vi "Convert Time to UTC String.vi"(11 "timestamp":timestamp) -> (3 "UTC string":string)   [LabVIEW 2019, in "CAN Stream Support Workspace Shared.lvlib"]
uses:
  CAN Stream Support Workspace Shared.lvlib
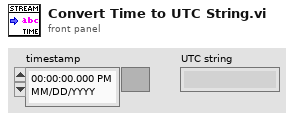
[diagram p1: front panel]
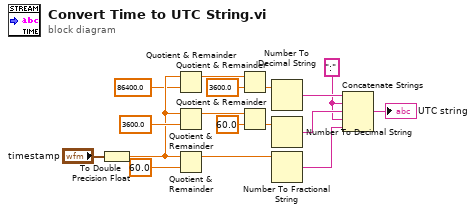
[diagram p0: block diagram]
diagram:
  w3 = ":" ("string")
  n1 = To Double Precision Float(number="timestamp") -> (double precision float=w14:dbl)
  n2 = Quotient & Remainder(x=w14, y=86400.0) -> (x-y*floor(x/y)=w10:dbl)  [unwired: 1 out]
  n3 = Quotient & Remainder(x=w14, y=3600.0) -> (x-y*floor(x/y)=w11:dbl)  [unwired: 1 out]
  n4 = Quotient & Remainder(x=w14, y=60.0) -> (x-y*floor(x/y)=w5:dbl)  [unwired: 1 out]
  n5 = Quotient & Remainder(x=w10, y=3600.0) -> (floor(x/y)=w9:dbl)  [unwired: 1 out]
  n6 = Quotient & Remainder(x=w11, y=60.0) -> (floor(x/y)=w6:dbl)  [unwired: 1 out]
  n7 = Number To Decimal String(number=w9) -> (decimal integer string=w8:string)  [unwired: 1 in]
  n8 = Number To Decimal String(number=w6) -> (decimal integer string=w7:string)  [unwired: 1 in]
  n9 = Number To Fractional String(number=w5) -> (F-format string=w4:string)  [unwired: 3 in]
  n10 = Concatenate Strings(w8, w3, w7, w3, w4) -> (→"UTC string":string)
